vi "自动测试类型1.vi"(10 "测试类型1选择?":bool) -> ()   [LabVIEW 2010]
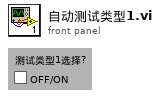
[diagram p1: front panel]
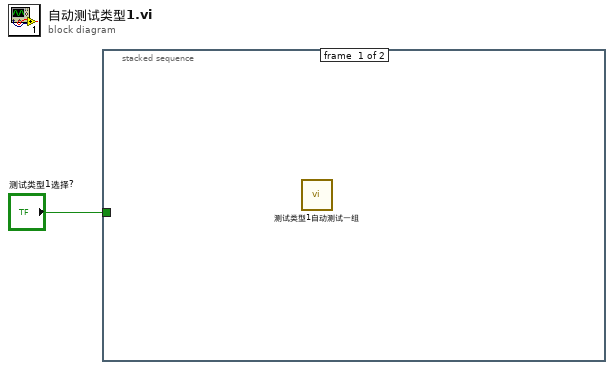
[diagram p0: block diagram]
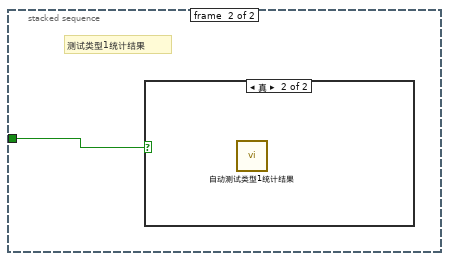
[diagram p2: hidden frame]
diagram:
  n1 = stacked-sequence {
    tunnel: "测试类型1选择?" -> [_ w2]
    frame #0 {
      n2 = call "测试类型1自动测试一组.vi"() -> ()  [unwired: 9 in]
    }
    frame #1 {
      # "测试类型1统计结果"
      n3 = case shown="真" w2 {
        frame False {
        }
        frame True {
          n4 = call "自动测试类型1统计结果.vi"() -> ()  [unwired: 12 in]
        }
      }
    }
  }
